vi "Facade.vi"(0 "Data In":T8, 2 "Display State In":T4 {"button state" items=["init", "not connect", "local disabled", "local hand", "set hand", "hand", "set auto", "auto", "dist"]}, 3 "Container State":T7) -> (6 "Data Out":T8, 7 "Display State Out":T4 {"button state" items=["init", "not connect", "local disabled", "local hand", "set hand", "hand", "set auto", "auto", "dist"]}, 8 "Action":T3)   [LabVIEW 2019, in "Heating.lvlib" / "Z_Hswitch_little.xctl"]
uses:
  Z_Hswitch_little.xctl
  Data.ctl
  <vilib>/_xctls/Container State.ctl
  State.ctl
  Z_source.ctl
  AutoButton_state.ctl
  <vilib>/_xctls/Action.ctl
  Z_HSwitch.ctl
  Y_SourceInd.ctl
  <vilib>/_xctls/XControlSupport.lvlib
  Timer Delay/Timers.lvlib
  Heating.lvlib
panel:
  in  "Z_HSwitch":T1
  out "Z1 ind":T2
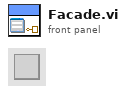
[diagram p1: front panel]
types:
  T1 = typedef "Heating.lvlib/Z_Hswitch_little.xctl/Z_HSwitch.ctl" = bool
  T2 = typedef "Heating.lvlib/Z_Hswitch_little.xctl/Y_SourceInd.ctl" = u8
  T3 = typedef "XControlSupport.lvlib/Action.ctl" = cluster{"Data Changed?":bool, "State Changed?":bool, "Action Name":string}
  T4 = typedef "Heating.lvlib/Z_Hswitch_little.xctl/State.ctl" = cluster{"Z_Source":cluster{"connect":bool, "Z_Source":T5}, "Write":bool, "Z1_ind":u8, "button state":T6, "reset_timer":bool, "load_timer":bool, "end_timer":bool}
  T5 = typedef "Heating.lvlib/Z_source.ctl" = enum8{"initialize", "local disabled", "local hand", "hand", "auto", "dist"}
  T6 = typedef "Heating.lvlib/Z_Hswitch_little.xctl/AutoButton_state.ctl" = u16
  T7 = typedef "XControlSupport.lvlib/Container State.ctl" = cluster{"Indicator?":bool, "Run Mode?":bool, " Refnum":refnum<vi>}
  T8 = typedef "Heating.lvlib/Z_Hswitch_little.xctl/Data.ctl" = bool
  T9 = enum8{"Enabled", "Disabled", "Disabled and Grayed Out"}
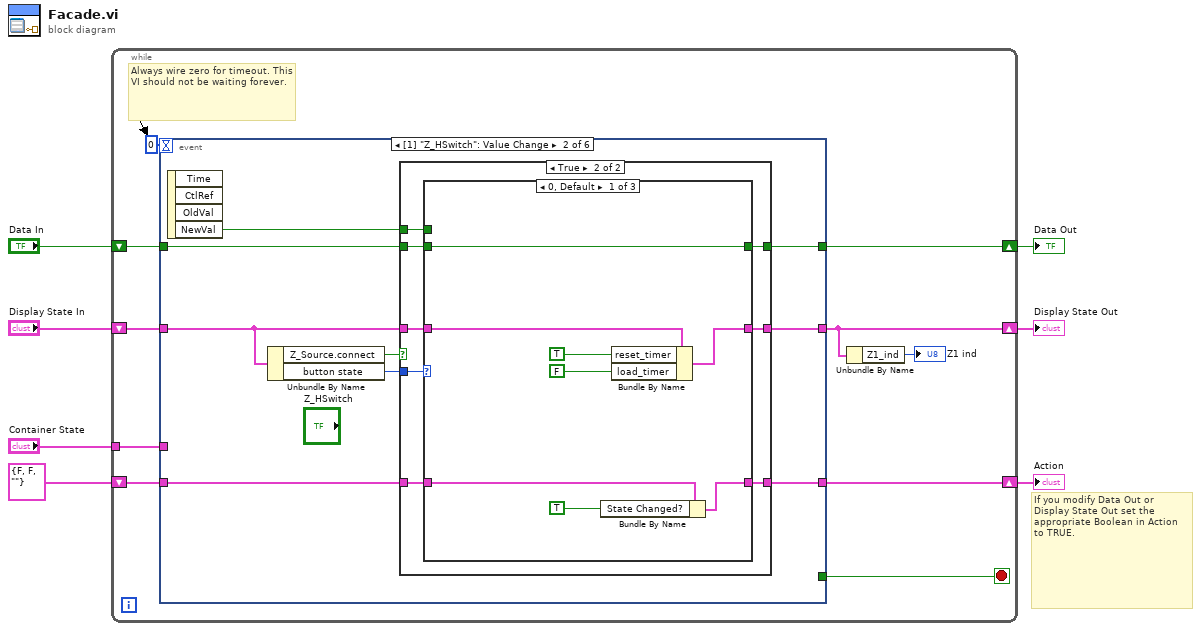
[diagram p0: block diagram]
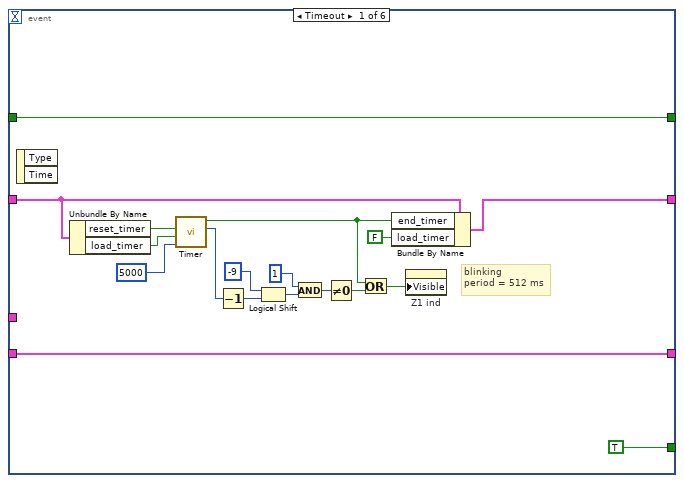
[diagram p2: hidden frame]
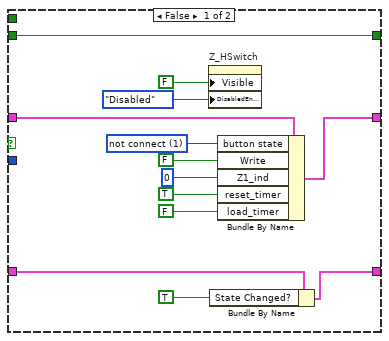
[diagram p3: hidden frame]
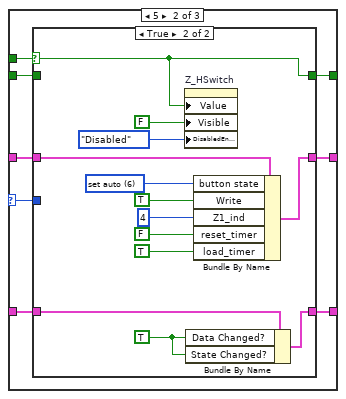
[diagram p4: hidden frame]
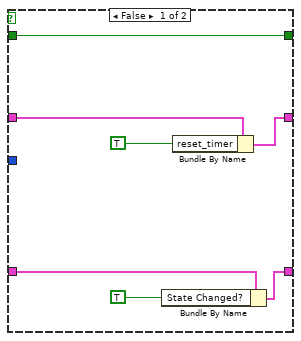
[diagram p5: hidden frame]
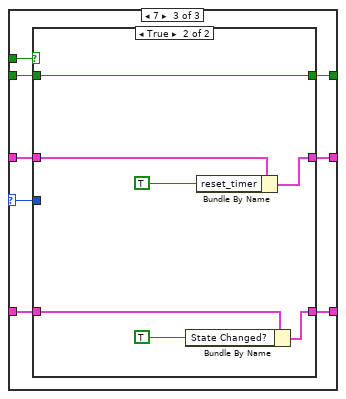
[diagram p6: hidden frame]
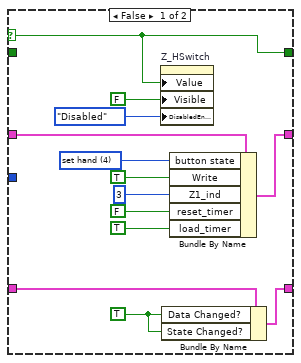
[diagram p7: hidden frame]
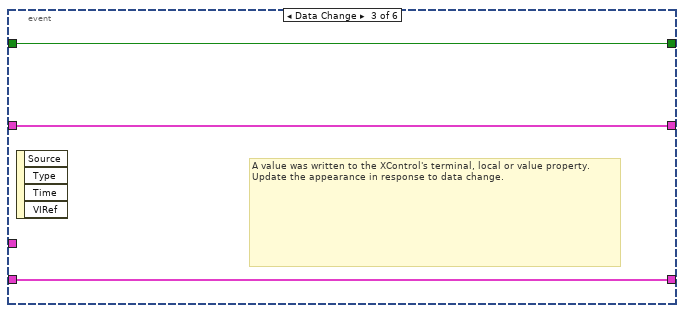
[diagram p8: hidden frame]
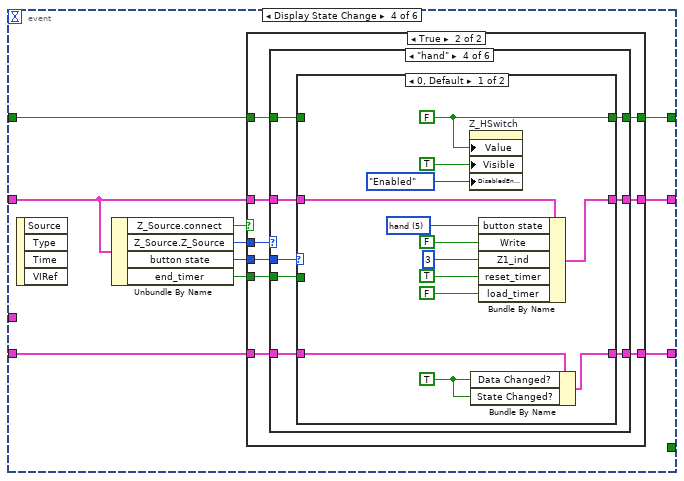
[diagram p9: hidden frame]
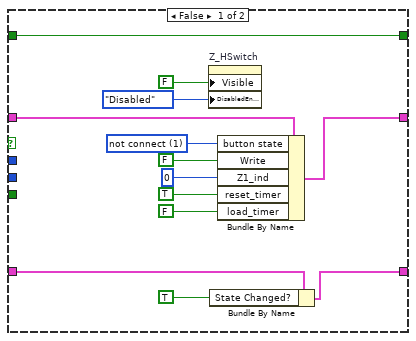
[diagram p10: hidden frame]
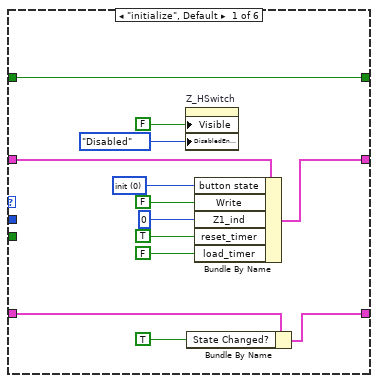
[diagram p11: hidden frame]
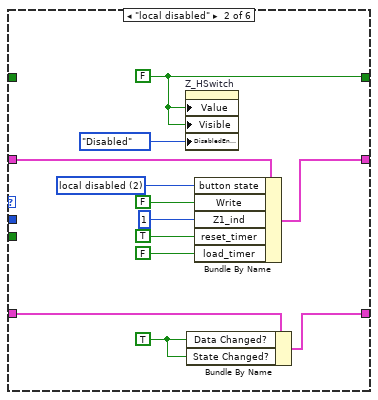
[diagram p12: hidden frame]
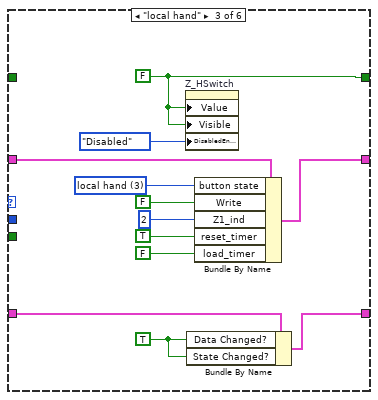
[diagram p13: hidden frame]
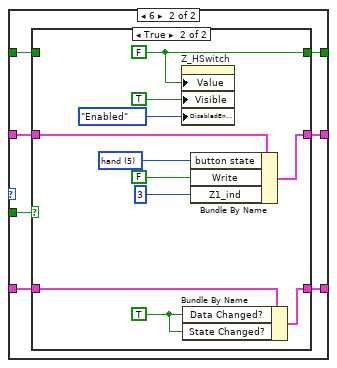
[diagram p14: hidden frame]
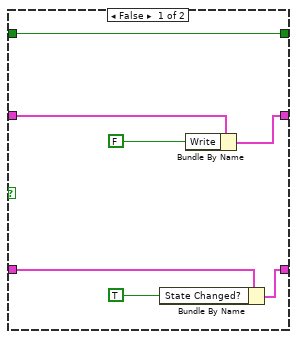
[diagram p15: hidden frame]
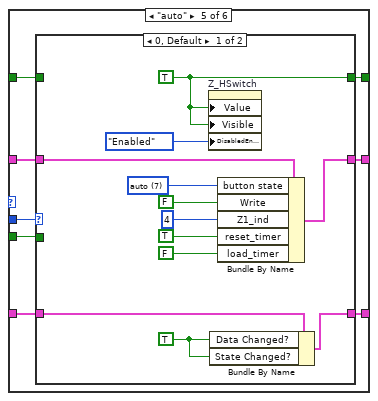
[diagram p16: hidden frame]
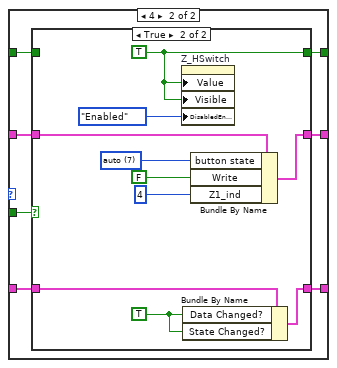
[diagram p17: hidden frame]
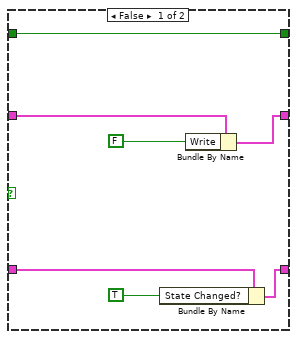
[diagram p18: hidden frame]
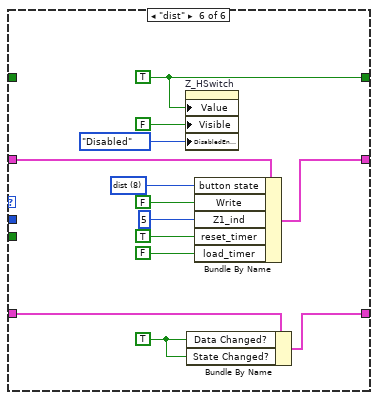
[diagram p19: hidden frame]
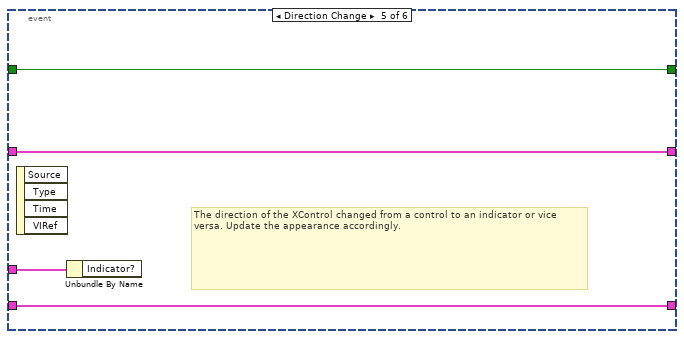
[diagram p20: hidden frame]
diagram:
  # "If you modify Data Out or\nDisplay State Out set the\nappropriate Boolean in Action\nto TRUE."
  n1 = while {
    shift-right: [w8] -> w4
    shift-left: "Display State In" -> [w17]
    tunnel: "Container State" -> [w14]
    shift-right: [w12] -> w7
    shift-left: "Data In" -> [w13]
    shift-right: [w10] -> w2
    shift-left: T3 {"Data Changed?"=FALSE, "State Changed?"=FALSE, "Action Name"=""} ("Action") -> [w11]
    stop <- w16 stop-if-true
    # "Always wire zero for timeout. This\nVI should not be waiting forever."
    n2 = event shown="[1] \"Z_HSwitch\": Value Change" {
      selector: _ -> [_ _ _ _ _ _]
      dyn-events: _ -> [_ _ _ _ _ _]
      timeout: 0 -> [_ _ _ _ _ _]
      tunnel: w17 -> [w30 w38 w131 w136 w307 w311]
      tunnel: [w29 w43 w131 w140 w307 w311] -> w8
      tunnel: [TRUE _ _ _ _ _] -> w16
      tunnel: w14 -> [_ _ _ _ w308 w312]
      tunnel: w13 -> [w33 w42 w132 w142 w306 w310]
      tunnel: [w33 w41 w132 w141 w306 w310] -> w12
      tunnel: [w34 w39 w130 w138 w305 w309] -> w10
      tunnel: w11 -> [w34 w40 w130 w139 w305 w309]
      event Timeout {
        # "blinking\nperiod = 512 ms"
        n3 = event-data() -> ()  [unwired: 1 in, 2 out]
        n4 = Unbundle By Name(w30) -> ("reset_timer"=w32:bool, "load_timer"=w31:bool)
        n5 = call "Timer.vi"("ms"=5000, "Load (F)"=w31, "Reset (F)"=w32) -> ("t ms"=w27:u32, "End"=w23:bool)  [unwired: 6 in]
        n6 = Decrement(x=w27) -> (x-1=w22:u32)
        n7 = Logical Shift(y=i16 -9, x=w22) -> (x << y=w20:u32)
        n8 = And(x=u32 1 ("y"), y=w20) -> (x .and. y?=w18:u32)
        n9 = Not Equal To 0?(x=w18) -> (x != 0?=w24:bool)
        n10 = Or(x=w23, y=w24) -> (x .or. y?=w25:bool)
        n11 = Bundle By Name(cluster=w30, "end_timer"=w23, "load_timer"=FALSE) -> (w29:T4)
        n12 = property on="Z1 ind" class="Ring (strict)"("Visible"=w25) -> ()  [unwired: 2 in, 2 out]
      }
      event Value Change {
        n13 = event-data() -> ("NewVal"=w44:T1)  [unwired: 1 in, 3 out]
        n14 = Unbundle By Name(w38) -> ("Z_Source.connect"=w37:bool, "button state"=w36:T6)
        n15 = case shown="True" w37 {
          tunnel: w36 -> [_ w65]
          tunnel: w44 -> [_ w64]
          tunnel: w38 -> [w52 w63]
          tunnel: [w51 w62] -> w43
          tunnel: w42 -> [w57 w61]
          tunnel: [w57 w60] -> w41
          tunnel: w40 -> [w49 w58]
          tunnel: [w48 w59] -> w39
          frame False {
            w53 = T6 1 items=["init", "not connect", "local disabled", "local hand", "set hand", "hand", "set auto", "auto", "dist"] ("f 3")
            n16 = property on="Z_HSwitch" class="Bool (strict)"("Visible"=FALSE ("Z_ASwitch"), "DisabledEnum"=T9."Disabled" ("Disabled")) -> ()  [unwired: 2 in, 2 out]
            n17 = Bundle By Name(cluster=w49, "State Changed?"=TRUE ("Data Changed?")) -> (w48:T3)
            n18 = Bundle By Name(cluster=w52, "button state"=w53, "Write"=FALSE ("Z_ASwitch"), "Z1_ind"=u8 0 ("Z1_ind visu"), "reset_timer"=TRUE ("Z_ASwitch"), "load_timer"=FALSE ("Z_ASwitch")) -> (w51:T4)
          }
          frame True {
            n19 = case shown="0, Default" w65 {
              selector: w65 -> [_ w80 w108]
              tunnel: w64 -> [_ w81 w109]
              tunnel: w63 -> [w72 w79 w107]
              tunnel: [w71 w78 w106] -> w62
              tunnel: w61 -> [w70 w76 w105]
              tunnel: [w70 w77 w104] -> w60
              tunnel: [w67 w74 w102] -> w59
              tunnel: w58 -> [w68 w75 w103]
              frame 0, Default {
                # "local hand"
                n20 = Bundle By Name(cluster=w68, "State Changed?"=TRUE ("Data Changed?")) -> (w67:T3)
                n21 = Bundle By Name(cluster=w72, "reset_timer"=TRUE, "load_timer"=FALSE) -> (w71:T4)
              }
              frame 5 {
                # "local hand"
                n22 = case shown="True" w81 {
                  selector: w81 -> [_ w93]
                  tunnel: w80 -> [_ _]
                  tunnel: w79 -> [w87 w95]
                  tunnel: [w86 w94] -> w78
                  tunnel: [w85 w93] -> w77
                  tunnel: w76 -> [w85 _]
                  tunnel: w75 -> [w83 w91]
                  tunnel: [w82 w90] -> w74
                  frame False {
                    n23 = Bundle By Name(cluster=w83, "State Changed?"=TRUE ("Data Changed?")) -> (w82:T3)
                    n24 = Bundle By Name(cluster=w87, "reset_timer"=TRUE) -> (w86:T4)
                  }
                  frame True {
                    w92 = TRUE ("Data Changed?")
                    w99 = T6 6 items=["init", "not connect", "local disabled", "local hand", "set hand", "hand", "set auto", "auto", "dist"] ("f 3")
                    n25 = property on="Z_HSwitch" class="Bool (strict)"("Value"=w93, "Visible"=FALSE ("Z_ASwitch"), "DisabledEnum"=T9."Disabled" ("Disabled")) -> ()  [unwired: 2 in, 2 out]
                    n26 = Bundle By Name(cluster=w91, "Data Changed?"=w92, "State Changed?"=w92) -> (w90:T3)
                    n27 = Bundle By Name(cluster=w95, "button state"=w99, "Write"=TRUE ("Z_ASwitch"), "Z1_ind"=u8 4 ("Z1_ind visu"), "reset_timer"=FALSE ("Z_ASwitch"), "load_timer"=TRUE ("Z_ASwitch")) -> (w94:T4)
                  }
                }
              }
              frame 7 {
                # "local hand"
                n28 = case shown="True" w109 {
                  selector: w109 -> [w114 _]
                  tunnel: w108 -> [_ _]
                  tunnel: w107 -> [w116 w128]
                  tunnel: [w115 w127] -> w106
                  tunnel: w105 -> [_ w129]
                  tunnel: [w114 w129] -> w104
                  tunnel: w103 -> [w112 w124]
                  tunnel: [w111 w123] -> w102
                  frame False {
                    w113 = TRUE ("Data Changed?")
                    w117 = T6 4 items=["init", "not connect", "local disabled", "local hand", "set hand", "hand", "set auto", "auto", "dist"] ("f 3")
                    n29 = property on="Z_HSwitch" class="Bool (strict)"("Value"=w114, "Visible"=FALSE ("Z_ASwitch"), "DisabledEnum"=T9."Disabled" ("Disabled")) -> ()  [unwired: 2 in, 2 out]
                    n30 = Bundle By Name(cluster=w112, "Data Changed?"=w113, "State Changed?"=w113) -> (w111:T3)
                    n31 = Bundle By Name(cluster=w116, "button state"=w117, "Write"=TRUE ("Z_ASwitch"), "Z1_ind"=u8 3 ("Z1_ind visu"), "reset_timer"=FALSE ("Z_ASwitch"), "load_timer"=TRUE ("Z_ASwitch")) -> (w115:T4)
                  }
                  frame True {
                    n32 = Bundle By Name(cluster=w124, "State Changed?"=TRUE ("Data Changed?")) -> (w123:T3)
                    n33 = Bundle By Name(cluster=w128, "reset_timer"=TRUE ("Z1_ind_blinking")) -> (w127:T4)
                  }
                }
              }
            }
          }
        }
      }
      event Data Change {
        # "A value was written to the XControl's terminal, local or value property.\nUpdate the appearance in response to data change."
        n34 = event-data() -> ()  [unwired: 1 in, 4 out]
      }
      event Display State Change {
        n35 = event-data() -> ()  [unwired: 1 in, 4 out]
        n36 = Unbundle By Name(w136) -> ("Z_Source.connect"=w137:bool, "Z_Source.Z_Source"=w134:T5, "button state"=w133:T6, "end_timer"=w135:bool)
        n37 = case shown="True" w137 {
          tunnel: w134 -> [_ w164]
          tunnel: w136 -> [w150 w163]
          tunnel: [w149 w162] -> w140
          tunnel: w142 -> [w155 w161]
          tunnel: [w155 w160] -> w141
          tunnel: w139 -> [w147 w158]
          tunnel: [w146 w159] -> w138
          tunnel: w135 -> [_ w157]
          tunnel: w133 -> [_ w156]
          frame False {
            w151 = T6 1 items=["init", "not connect", "local disabled", "local hand", "set hand", "hand", "set auto", "auto", "dist"] ("f 3")
            n38 = property on="Z_HSwitch" class="Bool (strict)"("Visible"=FALSE ("Z_ASwitch"), "DisabledEnum"=T9."Disabled" ("Disabled")) -> ()  [unwired: 2 in, 2 out]
            n39 = Bundle By Name(cluster=w147, "State Changed?"=TRUE ("Data Changed?")) -> (w146:T3)
            n40 = Bundle By Name(cluster=w150, "button state"=w151, "Write"=FALSE ("Z_ASwitch"), "Z1_ind"=u8 0 ("Z1_ind visu"), "reset_timer"=TRUE ("Z_ASwitch"), "load_timer"=FALSE ("Z_ASwitch")) -> (w149:T4)
          }
          frame True {
            n41 = case shown="\"hand\"" w164 {
              tunnel: w163 -> [w177 w189 w201 w206 w252 w304]
              tunnel: [w176 w188 w200 w208 w254 w303] -> w162
              tunnel: w161 -> [w166 _ _ w207 w253 _]
              tunnel: [w166 w179 w191 w209 w255 w293] -> w160
              tunnel: [w174 w186 w198 w202 w248 w301] -> w159
              tunnel: w158 -> [w175 w187 w199 w203 w249 w302]
              tunnel: w157 -> [_ _ _ w205 w251 _]
              tunnel: w156 -> [_ _ _ w204 w250 _]
              frame "initialize", Default {
                w171 = T6 0 items=["init", "not connect", "local disabled", "local hand", "set hand", "hand", "set auto", "auto", "dist"] ("f 3")
                # "local hand"
                n42 = property on="Z_HSwitch" class="Bool (strict)"("Visible"=FALSE ("Z_ASwitch"), "DisabledEnum"=T9."Disabled" ("Disabled")) -> ()  [unwired: 2 in, 2 out]
                n43 = Bundle By Name(cluster=w175, "State Changed?"=TRUE ("Data Changed?")) -> (w174:T3)
                n44 = Bundle By Name(cluster=w177, "button state"=w171, "Write"=FALSE ("Z_ASwitch"), "Z1_ind"=u8 0 ("Z1_ind visu"), "reset_timer"=TRUE ("Z_ASwitch"), "load_timer"=FALSE ("Z_ASwitch")) -> (w176:T4)
              }
              frame "local disabled" {
                w178 = TRUE ("Data Changed?")
                w179 = FALSE ("Z_ASwitch")
                w183 = T6 2 items=["init", "not connect", "local disabled", "local hand", "set hand", "hand", "set auto", "auto", "dist"] ("f 3")
                # "local hand"
                n45 = property on="Z_HSwitch" class="Bool (strict)"("Value"=w179, "Visible"=w179, "DisabledEnum"=T9."Disabled" ("Disabled")) -> ()  [unwired: 2 in, 2 out]
                n46 = Bundle By Name(cluster=w187, "Data Changed?"=w178, "State Changed?"=w178) -> (w186:T3)
                n47 = Bundle By Name(cluster=w189, "button state"=w183, "Write"=FALSE ("Z_ASwitch"), "Z1_ind"=u8 1 ("Z1_ind visu"), "reset_timer"=TRUE ("Z_ASwitch"), "load_timer"=FALSE ("Z_ASwitch")) -> (w188:T4)
              }
              frame "local hand" {
                w190 = TRUE ("Data Changed?")
                w191 = FALSE ("Z_ASwitch")
                w195 = T6 3 items=["init", "not connect", "local disabled", "local hand", "set hand", "hand", "set auto", "auto", "dist"] ("f 3")
                # "local hand"
                n48 = property on="Z_HSwitch" class="Bool (strict)"("Value"=w191, "Visible"=w191, "DisabledEnum"=T9."Disabled" ("Disabled")) -> ()  [unwired: 2 in, 2 out]
                n49 = Bundle By Name(cluster=w199, "Data Changed?"=w190, "State Changed?"=w190) -> (w198:T3)
                n50 = Bundle By Name(cluster=w201, "button state"=w195, "Write"=FALSE ("Z_ASwitch"), "Z1_ind"=u8 2 ("Z1_ind visu"), "reset_timer"=TRUE ("Z_ASwitch"), "load_timer"=FALSE ("Z_ASwitch")) -> (w200:T4)
              }
              frame "hand" {
                # "local hand"
                n51 = case shown="0, Default" w204 {
                  tunnel: w205 -> [_ w229]
                  tunnel: w206 -> [w219 w223]
                  tunnel: [w210 w224] -> w208
                  tunnel: w207 -> [_ w228]
                  tunnel: [w215 w227] -> w209
                  tunnel: w203 -> [w217 w225]
                  tunnel: [w216 w226] -> w202
                  frame 0, Default {
                    w211 = TRUE ("Data Changed?")
                    w215 = FALSE ("Z_ASwitch")
                    w220 = T6 5 items=["init", "not connect", "local disabled", "local hand", "set hand", "hand", "set auto", "auto", "dist"] ("f 3")
                    n52 = property on="Z_HSwitch" class="Bool (strict)"("Value"=w215, "Visible"=TRUE ("Z_ASwitch"), "DisabledEnum"=T9."Enabled" ("Disabled")) -> ()  [unwired: 2 in, 2 out]
                    n53 = Bundle By Name(cluster=w217, "Data Changed?"=w211, "State Changed?"=w211) -> (w216:T3)
                    n54 = Bundle By Name(cluster=w219, "button state"=w220, "Write"=FALSE ("Z_ASwitch"), "Z1_ind"=u8 3 ("Z1_ind visu"), "reset_timer"=TRUE ("Z_ASwitch"), "load_timer"=FALSE ("Z_ASwitch")) -> (w210:T4)
                  }
                  frame 6 {
                    n55 = case shown="True" w229 {
                      tunnel: w223 -> [w236 w247]
                      tunnel: [w235 w246] -> w224
                      tunnel: w228 -> [w231 _]
                      tunnel: [w231 w239] -> w227
                      tunnel: [w233 w244] -> w226
                      tunnel: w225 -> [w234 w245]
                      frame False {
                        # "local hand"
                        n56 = Bundle By Name(cluster=w234, "State Changed?"=TRUE ("Data Changed?")) -> (w233:T3)
                        n57 = Bundle By Name(cluster=w236, "Write"=FALSE ("Z_ASwitch")) -> (w235:T4)
                      }
                      frame True {
                        w241 = TRUE ("Data Changed?")
                        w239 = FALSE ("Z_ASwitch")
                        w238 = T6 5 items=["init", "not connect", "local disabled", "local hand", "set hand", "hand", "set auto", "auto", "dist"] ("f 3")
                        # "local hand"
                        n58 = property on="Z_HSwitch" class="Bool (strict)"("Value"=w239, "Visible"=TRUE ("Z_ASwitch"), "DisabledEnum"=T9."Enabled" ("Disabled")) -> ()  [unwired: 2 in, 2 out]
                        n59 = Bundle By Name(cluster=w245, "Data Changed?"=w241, "State Changed?"=w241) -> (w244:T3)
                        n60 = Bundle By Name(cluster=w247, "button state"=w238, "Write"=FALSE ("Z_ASwitch"), "Z1_ind"=u8 3 ("Z1_ind visu")) -> (w246:T4)
                      }
                    }
                  }
                }
              }
              frame "auto" {
                # "local hand"
                n61 = case shown="0, Default" w250 {
                  tunnel: w251 -> [_ w274]
                  tunnel: w252 -> [w264 w273]
                  tunnel: [w263 w272] -> w254
                  tunnel: w253 -> [_ w271]
                  tunnel: [w259 w270] -> w255
                  tunnel: w249 -> [w261 w268]
                  tunnel: [w260 w269] -> w248
                  frame 0, Default {
                    w256 = TRUE ("Data Changed?")
                    w259 = TRUE ("Z_ASwitch")
                    w265 = T6 7 items=["init", "not connect", "local disabled", "local hand", "set hand", "hand", "set auto", "auto", "dist"] ("f 3")
                    n62 = property on="Z_HSwitch" class="Bool (strict)"("Value"=w259, "Visible"=w259, "DisabledEnum"=T9."Enabled" ("Disabled")) -> ()  [unwired: 2 in, 2 out]
                    n63 = Bundle By Name(cluster=w261, "Data Changed?"=w256, "State Changed?"=w256) -> (w260:T3)
                    n64 = Bundle By Name(cluster=w264, "button state"=w265, "Write"=FALSE ("Z_ASwitch"), "Z1_ind"=u8 4 ("Z1_ind visu"), "reset_timer"=TRUE ("Z_ASwitch"), "load_timer"=FALSE ("Z_ASwitch")) -> (w263:T4)
                  }
                  frame 4 {
                    n65 = case shown="True" w274 {
                      tunnel: w273 -> [w281 w291]
                      tunnel: [w280 w290] -> w272
                      tunnel: w271 -> [w276 _]
                      tunnel: [w276 w282] -> w270
                      tunnel: [w278 w288] -> w269
                      tunnel: w268 -> [w279 w289]
                      frame False {
                        # "local hand"
                        n66 = Bundle By Name(cluster=w279, "State Changed?"=TRUE ("Data Changed?")) -> (w278:T3)
                        n67 = Bundle By Name(cluster=w281, "Write"=FALSE ("Z_ASwitch")) -> (w280:T4)
                      }
                      frame True {
                        w283 = TRUE ("Data Changed?")
                        w282 = TRUE ("Z_ASwitch")
                        w284 = T6 7 items=["init", "not connect", "local disabled", "local hand", "set hand", "hand", "set auto", "auto", "dist"] ("f 3")
                        # "local hand"
                        n68 = property on="Z_HSwitch" class="Bool (strict)"("Value"=w282, "Visible"=w282, "DisabledEnum"=T9."Enabled" ("Disabled")) -> ()  [unwired: 2 in, 2 out]
                        n69 = Bundle By Name(cluster=w289, "Data Changed?"=w283, "State Changed?"=w283) -> (w288:T3)
                        n70 = Bundle By Name(cluster=w291, "button state"=w284, "Write"=FALSE ("Z_ASwitch"), "Z1_ind"=u8 4 ("Z1_ind visu")) -> (w290:T4)
                      }
                    }
                  }
                }
              }
              frame "dist" {
                w293 = TRUE ("Z_ASwitch")
                w292 = TRUE ("Data Changed?")
                w298 = T6 8 items=["init", "not connect", "local disabled", "local hand", "set hand", "hand", "set auto", "auto", "dist"] ("f 3")
                # "local hand"
                n71 = property on="Z_HSwitch" class="Bool (strict)"("Value"=w293, "Visible"=FALSE ("Z_ASwitch"), "DisabledEnum"=T9."Disabled" ("Disabled")) -> ()  [unwired: 2 in, 2 out]
                n72 = Bundle By Name(cluster=w302, "Data Changed?"=w292, "State Changed?"=w292) -> (w301:T3)
                n73 = Bundle By Name(cluster=w304, "button state"=w298, "Write"=FALSE ("Z_ASwitch"), "Z1_ind"=u8 5 ("Z1_ind visu"), "reset_timer"=TRUE ("Z_ASwitch"), "load_timer"=FALSE ("Z_ASwitch")) -> (w303:T4)
              }
            }
          }
        }
      }
      event Direction Change {
        # "The direction of the XControl changed from a control to an indicator or vice versa. Update the appearance accordingly."
        n74 = event-data() -> ()  [unwired: 1 in, 4 out]
        n75 = Unbundle By Name(w308) -> ()  [unwired: 1 out]
      }
      event Exec State Change {
        # "The VI owning the XControl changed from Edit Mode  to Run Mode or vice versa.\nUpdate the appearance accordingly."
        # "Handle Edit Mode & Run Mode\ncase differently"
        n76 = event-data() -> ()  [unwired: 1 in, 4 out]
        n77 = Unbundle By Name(w312) -> ()  [unwired: 1 out]
      }
    }
    n78 = Unbundle By Name(w8) -> ("Z1_ind"=→"Z1 ind":u8)
  }
  "Display State Out" <- w4
  "Data Out" <- w7
  "Action" <- w2
